vi "LS350-Open_connection.vi"() -> (0 "error out":errorcluster, 1 "VISA resource name out":refnum<visa-resource-name>)   [LabVIEW 2019]
uses:
  Instrument_Setup.vi
panel:
  out "VISA resource name 3":refnum<visa-resource-name>
  in  "error in (no error)":errorcluster
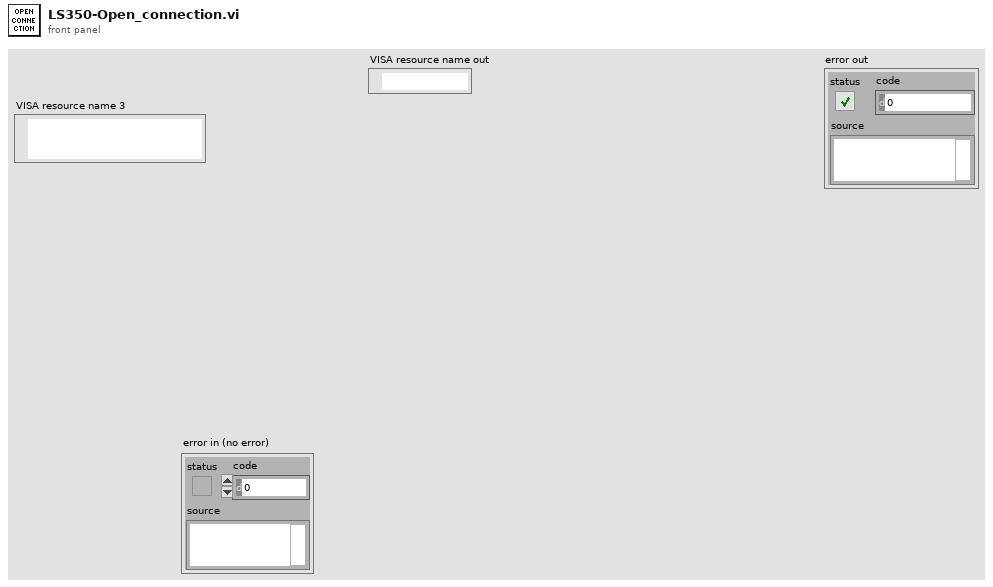
[diagram p1: front panel]
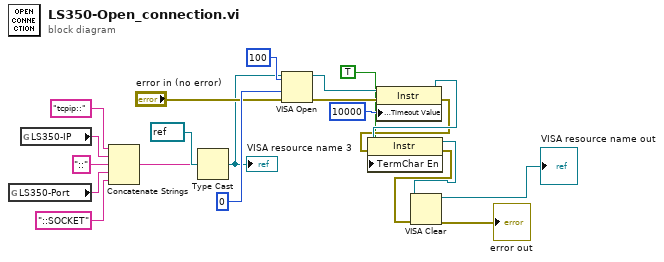
[diagram p0: block diagram]
diagram:
  n1 = global read "Instrument_Setup.vi" "LS350-Port"() -> (w6:string)
  n2 = global read "Instrument_Setup.vi" "LS350-IP"() -> (w7:string)
  n3 = Concatenate Strings("tcpip::" ("string"), w7, "::", w6, "::SOCKET") -> (w14:string)
  n4 = Type Cast(type=refnum<visa-resource-name> refnum ("VISA resource name"), x=w14) -> (*(type *) &x=w10:refnum<visa-resource-name>)
  "VISA resource name 3" <- w10
  n5 = VISA Open(timeout (0)=u32 100 ("VISA Open timeout (0)"), access mode=u32 0, error in (no error)="error in (no error)", VISA resource name=w10) -> (VISA resource name=w19:refnum<visa-resource-name>, error out=w11:errorcluster)  [unwired: 1 in]
  n6 = property class="Instr"(reference=w19, error in=w11, "General Settings:Timeout Value"=u32 10000) -> (reference out=w18:refnum<visa-resource-name>, error out=w17:errorcluster)
  n7 = property class="Instr"(reference=w18, error in=w17, "TermChar En"=TRUE) -> (reference out=w4:refnum<visa-resource-name>, error out=w3:errorcluster)
  n8 = VISA Clear(VISA resource name=w4, error in (no error)=w3) -> (VISA resource name out=→"VISA resource name out":refnum<visa-resource-name>, error out=→"error out":errorcluster)
